vi "onTestDiscovery.vi"(8 "error in (no error)":errorcluster, 11 "DMC Test Runner in":refnum<class "DMC Test Runner.lvclass">) -> (0 "error out":errorcluster, 2 "Tests VIs":path[](array[path]), 3 "DMC Test Runner out":refnum<class "DMC Test Runner.lvclass">)   [LabVIEW 2023, in "DMC Test Runner.lvclass"]
doc: "Searches the paths list for all VIs to run Unit Tests against.\nIf a VI path, checks bookmarks against VI.\nIf a directory, finds all VIs, checks for bookmarks.\nIf a LabVIEW project, find all VIs, checks for bookmarks."
uses:
  DMC Test Runner.lvclass
  DMC Test Runner.lvclass/DMC Test Runner.ctl
  071921aa-1ecc-45f1-a4fd-f8c74b4d2d4d.vi
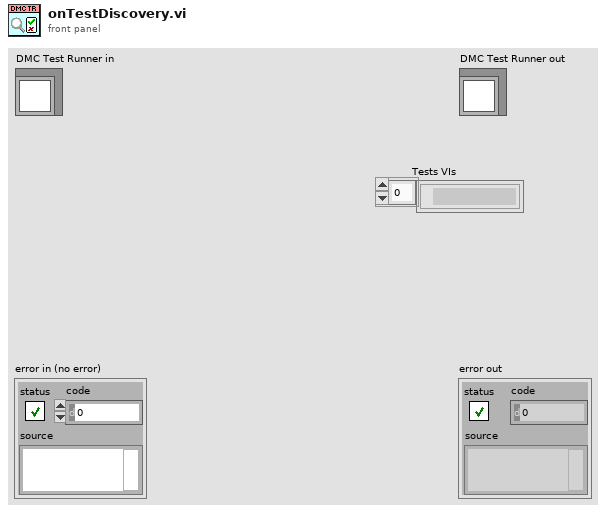
[diagram p1: front panel]
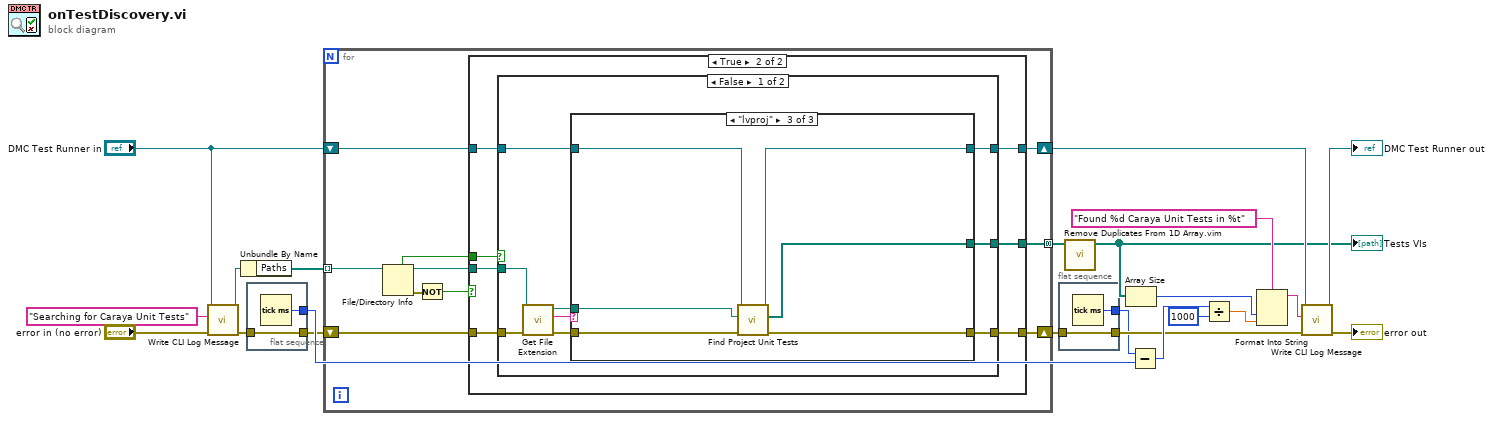
[diagram p0: block diagram]
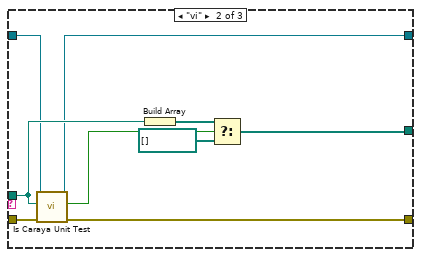
[diagram p4: hidden frame]
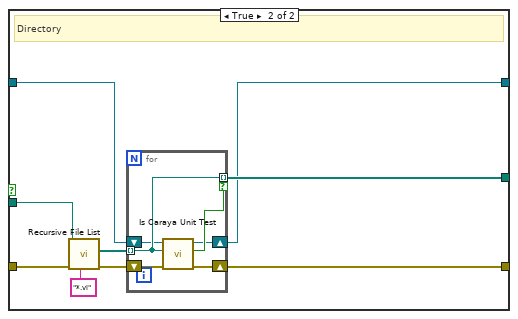
[diagram p5: hidden frame]
diagram:
  n1 = call "Write CLI Log Message.vi"("error in (no error)"="error in (no error)", "Message"="Searching for Caraya Unit Tests", "DMC Test Runner in"="DMC Test Runner in") -> ("error out"=w4:errorcluster, "DMC Test Runner out"=w20:refnum<class "DMC Test Runner.lvclass">)  [unwired: 7 in]
  n2 = Unbundle By Name(w20) -> ("Paths"=w22:path[])
  n3 = flat-sequence {
    tunnel: [w24] -> w6
    tunnel: [w23] -> w5
    tunnel: w4 -> [w23]
    frame #0 {
      n4 = Tick Count (ms)() -> (millisecond timer value=w24:u32)
    }
  }
  n5 = for {
    shift-right: [w34] -> w3
    shift-left: w5 -> [w33]
    tunnel: w22 -> [w25] mode=indexing
    shift-right: [w32] -> w15
    shift-left: "DMC Test Runner in" -> [w31]
    tunnel: [w30] -> w17 mode=concatenating
    n6 = File/Directory Info(path=w25) -> (path out=w26:path, directory=w28:bool, error out=w27:errorcluster)  [unwired: 1 in, 4 out]
    n7 = Not(x=w27) -> (.not. x?=w29:bool)
    n8 = case shown="True" w29 {
      tunnel: [w36 w42] -> w34
      tunnel: w33 -> [w36 w41]
      tunnel: w26 -> [_ w40]
      tunnel: w28 -> [_ w43]
      tunnel: [w35 w38] -> w32
      tunnel: w31 -> [w35 w37]
      tunnel: [_ w39] -> w30
      frame False {
      }
      frame True {
        n9 = case shown="False" w43 {
          tunnel: [w47 w72] -> w42
          tunnel: w41 -> [w52 w77]
          tunnel: w40 -> [w51 w76]
          tunnel: [w46 w73] -> w39
          tunnel: [w45 w71] -> w38
          tunnel: w37 -> [w44 w70]
          frame False {
            n10 = call <vilib>:"Get File Extension.vi"("error in (no error)"=w52, "file"=w51) -> ("error out"=w50:errorcluster, "lowercase file extension"=w49:string, "dup file"=w48:path)  [unwired: 5 in, 2 out]
            n11 = case shown="\"lvproj\"" w49 {
              tunnel: w50 -> [w54 w63 w69]
              tunnel: w48 -> [_ w58 w66]
              tunnel: [w54 w62 w64] -> w47
              tunnel: [_ w60 w65] -> w46
              tunnel: [w53 w56 w67] -> w45
              tunnel: w44 -> [w53 w55 w68]
              frame Default {
              }
              frame "vi" {
                n12 = call "Is Caraya Unit Test.vi"("Error in"=w63, "VI Path"=w58, "DMC Test Runner in"=w55) -> ("Error out"=w62:errorcluster, "Contains Define Test.vi?"=w57:bool, "DMC Test Runner out"=w56:refnum<class "DMC Test Runner.lvclass">)  [unwired: 6 in]
                n13 = Build Array(w58) -> (w61:path[])
                n14 = Select(t=w61, s=w57, f=path[] []) -> (s? t:f=w60:path[])
              }
              frame "lvproj" {
                n15 = call "Find Project Unit Tests.vi"("error in (no error)"=w69, "LabVIEW Project Path"=w66, "DMC Test Runner in"=w68) -> ("error out"=w64:errorcluster, "Caraya Unit Tests"=w65:path[], "DMC Test Runner out"=w67:refnum<class "DMC Test Runner.lvclass">)  [unwired: 6 in]
              }
            }
          }
          frame True {
            # "Directory"
            n16 = call <vilib>:"Recursive File List.vi"("pattern"="*.vi", "error in (no error)"=w77, "Folder Path"=w76) -> ("error out"=w74:errorcluster, "All Files in Dir"=w75:path[])  [unwired: 4 in, 3 out]
            n17 = for {
              tunnel: w75 -> [w82] mode=indexing
              tunnel: [w82] -> w73 mode=indexing if=w81
              shift-right: [w83] -> w72
              shift-left: w74 -> [w84]
              shift-right: [w79] -> w71
              shift-left: w70 -> [w80]
              n18 = call "Is Caraya Unit Test.vi"("Error in"=w84, "VI Path"=w82, "DMC Test Runner in"=w80) -> ("Error out"=w83:errorcluster, "Contains Define Test.vi?"=w81:bool, "DMC Test Runner out"=w79:refnum<class "DMC Test Runner.lvclass">)  [unwired: 6 in]
            }
          }
        }
      }
    }
  }
  n19 = flat-sequence {
    tunnel: [w86] -> w1
    tunnel: [w85] -> w2
    tunnel: w3 -> [w85]
    frame #0 {
      n20 = Tick Count (ms)() -> (millisecond timer value=w86:u32)
    }
  }
  n21 = call "Remove Duplicates From 1D Array.vim"("array"=w17) -> ("array with duplicates removed"=w9:path[])  [unwired: 10 in]
  "Tests VIs" <- w9
  n22 = Array Size(array=w9) -> (size(s)=w13:i32)
  n23 = Subtract(x=w1, y=w6) -> (x-y=w7:u32)
  n24 = Divide(x=w7, y=u32 1000) -> (x/y=w11:dbl)
  n25 = Format Into String(format string="Found %d Caraya Unit Tests in %t", w13, w11) -> (resulting string=w8:string)  [unwired: 2 in, 1 out]
  n26 = call "Write CLI Log Message.vi"("error in (no error)"=w2, "Message"=w8, "DMC Test Runner in"=w15) -> ("error out"=→"error out":errorcluster, "DMC Test Runner out"=→"DMC Test Runner out":refnum<class "DMC Test Runner.lvclass">)  [unwired: 7 in]
